vi "Between unit test.vi"(6 "x+y":dbl, 7 "String":string, 8 "entrée d'erreur (pas d'erreur)":errorcluster, 9 "x+y 2":dbl, 10 "Label":string, 11 "String 2":string) -> (0 "sortie d'erreur":errorcluster)   [LabVIEW 2021]
uses:
  <vilib>/addons/_JKI Toolkits/Caraya/classes/Properties.Assert/Properties.Assert.lvclass
  C:/Program Files (x86)/National Instruments/LabVIEW 2021/vi.lib/addons/_JKI Toolkits/Caraya/classes/Properties/Properties.lvclass
  <vilib>/addons/_JKI Toolkits/Caraya/classes/Assert/Assert True.vi
  <vilib>/addons/_JKI Toolkits/Caraya/classes/Assert/Assert.lvclass
  <vilib>/addons/_JKI Toolkits/Caraya/classes/Properties/Properties.lvclass
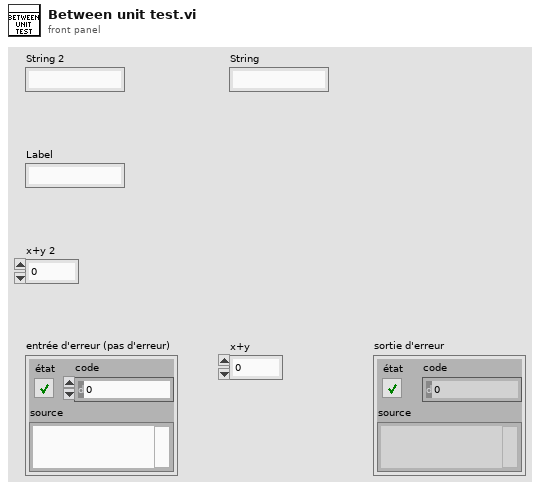
[diagram p1: front panel]
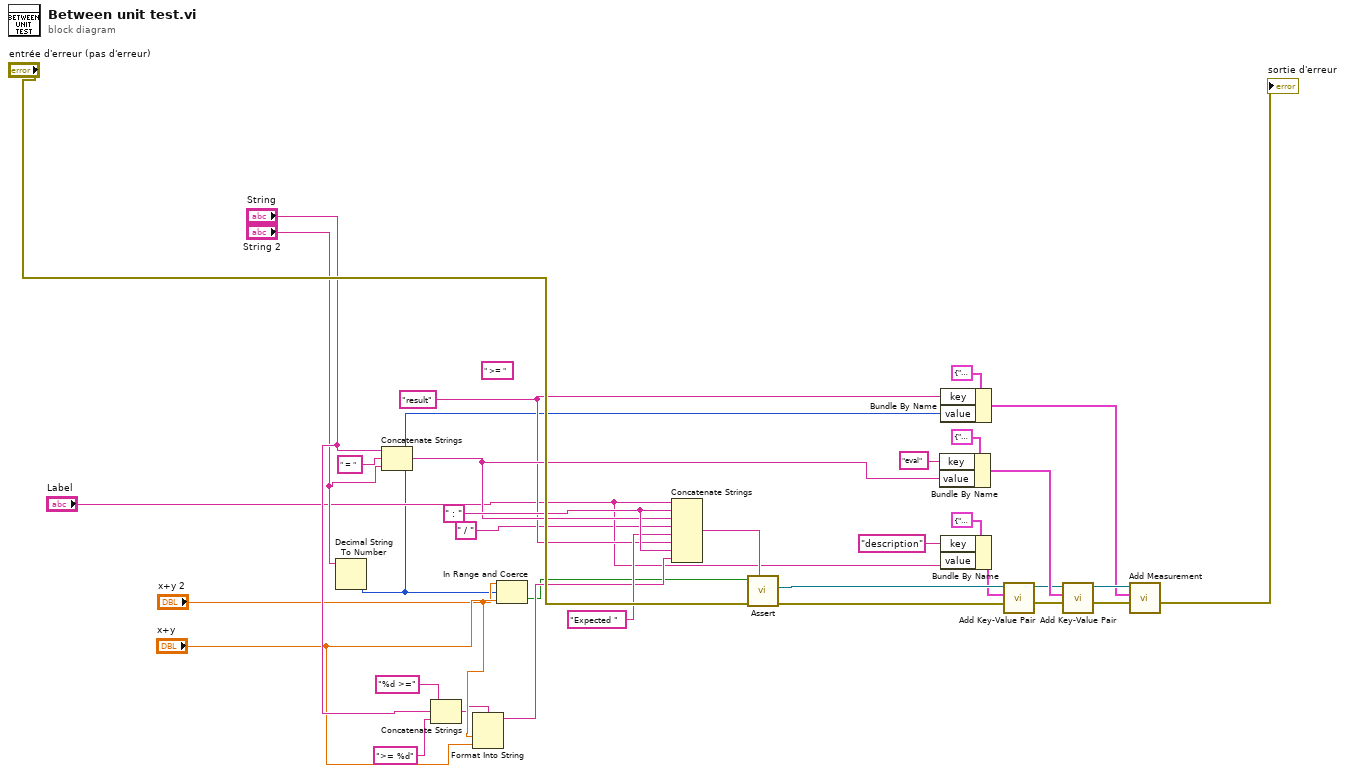
[diagram p0: block diagram]
diagram:
  w32 = " : " ("chaîne")
  (unwired) " >= " ("chaîne")
  w21 = "result"
  n1 = Decimal String To Number(string="String 2") -> (number=w17:i32)  [unwired: 2 in, 1 out]
  n2 = Concatenate Strings("String", " = " ("chaîne"), "String 2") -> (w30:string)
  n3 = Concatenate Strings("%d >=" ("chaîne"), "String", ">= %d" ("chaîne")) -> (w22:string)
  n4 = Format Into String(format string=w22, "x+y 2", "x+y") -> (resulting string=w27:string)  [unwired: 2 in, 1 out]
  n5 = In Range and Coerce(upper limit="x+y 2", x=w17, lower limit="x+y") -> (In Range?=w1:bool)  [unwired: 1 out]
  n6 = Concatenate Strings("Label", w32, w30, " / " ("chaîne"), "Expected " ("chaîne"), w21, w32, w27) -> (w20:string)
  n7 = call-poly <vilib>:"Assert.vi"("Label"=w20, "error in (no error)"="entrée d'erreur (pas d'erreur)", "True?"=w1) -> ("error out"=w14:errorcluster, "Properties"=w15:refnum<class "Properties.Assert.lvclass">)  [unwired: 7 in]
  n8 = Bundle By Name(cluster=cluster{"key":string, "value":variant} {"key"="", "value"=variant} ("entry"), "key"="eval", "value"=w30) -> (w12:cluster{"key":string, "value":variant})
  n9 = Bundle By Name(cluster=cluster{"key":string, "value":variant} {"key"="", "value"=variant} ("entry"), "key"=w21, "value"=w17) -> (w6:cluster{"key":string, "value":variant})
  n10 = Bundle By Name(cluster=cluster{"key":string, "value":variant} {"key"="", "value"=variant} ("entry"), "key"="description", "value"="Label") -> (w3:cluster{"key":string, "value":variant})
  n11 = call <vilib>:"Add Key-Value Pair.vi"("error in (no error)"=w14, "entry"=w3, "Properties in"=w15) -> ("error out"=w7:errorcluster, "Properties out"=w9:refnum<class "Properties.Assert.lvclass">)  [unwired: 7 in]
  n12 = call <vilib>:"Add Key-Value Pair.vi"("error in (no error)"=w7, "entry"=w12, "Properties in"=w9) -> ("error out"=w8:errorcluster, "Properties out"=w10:refnum<class "Properties.Assert.lvclass">)  [unwired: 7 in]
  n13 = call <vilib>:"Add Measurement.vi"("error in (no error)"=w8, "entry"=w6, "Properties"=w10) -> ("error out"=→"sortie d'erreur":errorcluster)  [unwired: 7 in, 1 out]
